vi "Update Category Name.vi"(8 "error in (no error)":errorcluster, 9 "Name":string, 10 "ID":i32, 11 "Database in":refnum<class "Database.lvclass">) -> (0 "error out":errorcluster, 3 "Database out":refnum<class "Database.lvclass">)   [LabVIEW 2018, in "Database.lvclass"]
uses:
  Database.lvclass
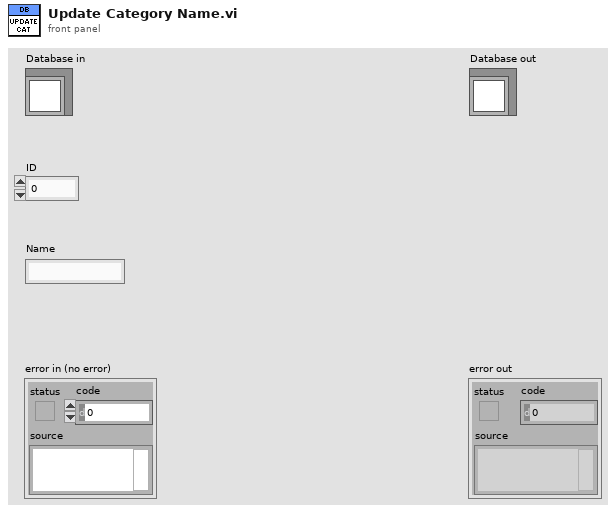
[diagram p1: front panel]
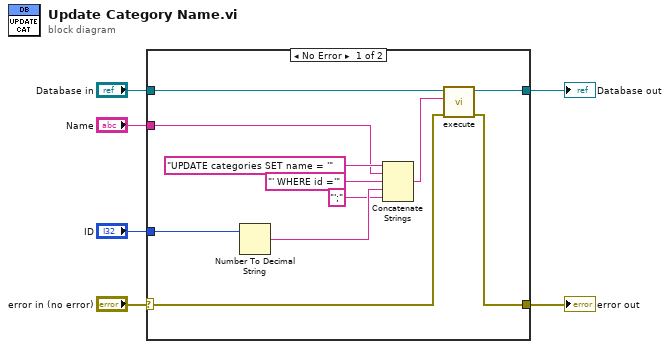
[diagram p0: block diagram]
diagram:
  n1 = case shown="No Error" "error in (no error)" {
    selector: "error in (no error)" -> [w7 w18]
    tunnel: "Database in" -> [w12 w19]
    tunnel: [w11 w19] -> w5
    tunnel: [w10 w18] -> w4
    tunnel: "Name" -> [w9 _]
    tunnel: "ID" -> [w8 _]
    frame No Error {
      n2 = Number To Decimal String(number=w8) -> (decimal integer string=w15:string)  [unwired: 1 in]
      n3 = Concatenate Strings("UPDATE categories SET name = '", w9, "' WHERE id ='", w15, "';") -> (w17:string)
      n4 = call "execute.vi"("error in (no error)"=w7, "SQL query"=w17, "Database in"=w12) -> ("error out"=w10:errorcluster, "Database out"=w11:refnum<class "Database.lvclass">)  [unwired: 7 in]
    }
    frame Error {
    }
  }
  "error out" <- w4
  "Database out" <- w5
